vi "PCT_FGV_Queue.vi"(7 "CMD":T1=enum."SET", 8 "error in (no error)":errorcluster) -> (0 "error out":errorcluster, 3 "Message Queues out":T2)   [LabVIEW 2020]
uses:
  Message Queue/All Message Queues.ctl
  Message Queue/Message Cluster.ctl
  PCT FGV CMD.ctl
  Message Queue/Message Queue.lvlib
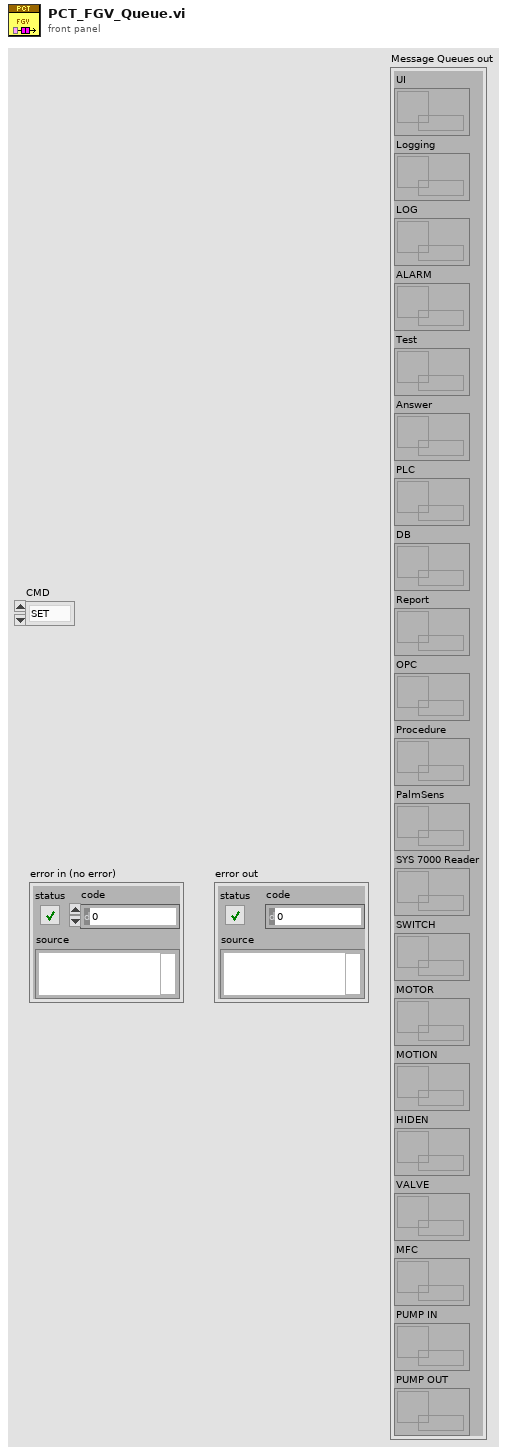
[diagram p1: front panel]
types:
  T1 = typedef "PCT FGV CMD.ctl" = enum16{"INIT", "GET", "SET"}
  T2 = typedef "Message Queue.lvlib/All Message Queues.ctl" = cluster{"UI":refnum<queue>, "Logging":refnum<queue>, "LOG":refnum<queue>, "ALARM":refnum<queue>, "Test":refnum<queue>, "Answer":refnum<queue>, "PLC":refnum<queue>, "DB":refnum<queue>, "Report":refnum<queue>, "OPC":refnum<queue>, "Procedure":refnum<queue>, "PalmSens":refnum<queue>, "SYS 7000 Reader":refnum<queue>, "SWITCH":refnum<queue>, "MOTOR":refnum<queue>, "MOTION":refnum<queue>, "HIDEN":refnum<queue>, "VALVE":refnum<queue>, "MFC":refnum<queue>, "PUMP IN":refnum<queue>, "PUMP OUT":refnum<queue>}
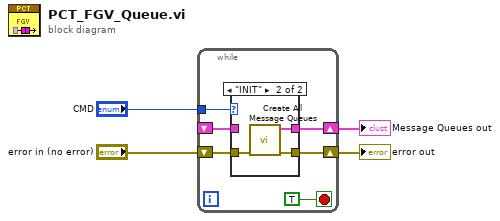
[diagram p0: block diagram]
diagram:
  n1 = while {
    shift-right: [w10] -> w4
    shift-left: "error in (no error)" -> [w9]
    tunnel: "CMD" -> [w8]
    shift-right: [w7] -> w1
    shift-left: _ -> [w6]
    stop <- TRUE stop-if-true
    n2 = case shown="\"INIT\"" w8 {
      tunnel: [w11 w15] -> w10
      tunnel: [w12 w14] -> w7
      tunnel: w9 -> [w11 w13]
      tunnel: w6 -> [w12 _]
      frame "GET", Default {
      }
      frame "INIT" {
        n3 = call "Create All Message Queues.vi"("error in (no error)"=w13) -> ("error out"=w15:errorcluster, "Message Queues out"=w14:T2)  [unwired: 9 in]
      }
    }
  }
  "error out" <- w4
  "Message Queues out" <- w1
